vi "Is Visible.vi"(8 "error in":errorcluster, 11 "type str":string) -> (0 "error out":errorcluster, 3 "yes":bool)   [LabVIEW 2014, in "lvprj2html.lvlib"]
uses:
  lvprj2html.lvlib
  <vilib>/regexp/Match Regular Expression.xnode
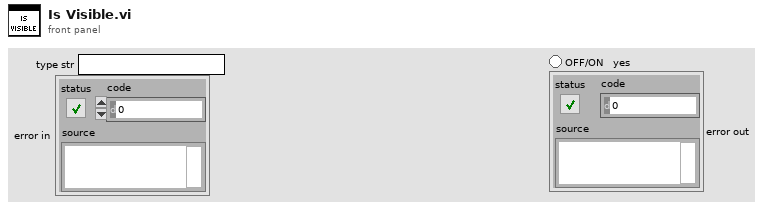
[diagram p1: front panel]
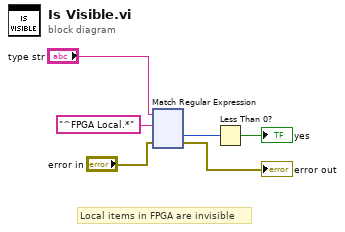
[diagram p0: block diagram]
diagram:
  # "Local items in FPGA are invisible"
  n1 = xnode "Match Regular Expression"("input string"="type str", "regular expression"="^FPGA Local.*", "error in"="error in") -> ("offset past match"=w2:i32, "error out"=→"error out":errorcluster)  [unwired: 3 in, 3 out]
  n2 = Less Than 0?(x=w2) -> (x < 0?=→"yes":bool)
